vi "Statemachine example.vi"() -> ()   [LabVIEW 2026]
uses:
  statemachine control_1.ctl
panel:
  out "motor on time[ms]":u32
  out "millisecond timer value":u32
  out "motor on":bool
  in  "MOTOR TIMER [ms]":i32
  in  "user button":bool
  in  "index pulse":bool
  out "State":T1
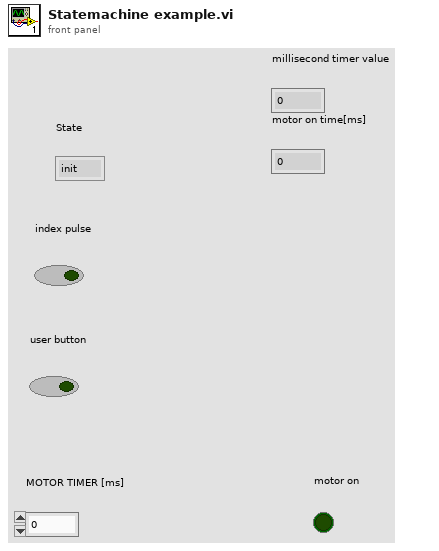
[diagram p1: front panel]
types:
  T1 = typedef "statemachine control_1.ctl" = enum16{"init", "waiting for pulse", "waiting for button", " running motor", "shut down"}
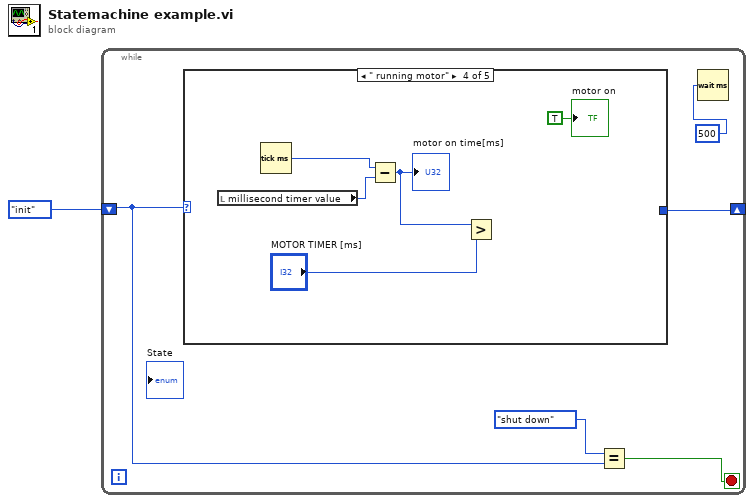
[diagram p0: block diagram]
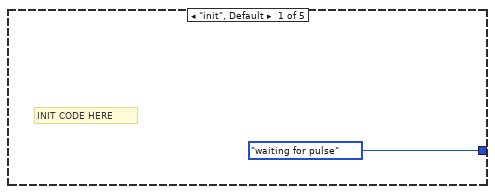
[diagram p2: hidden frame]
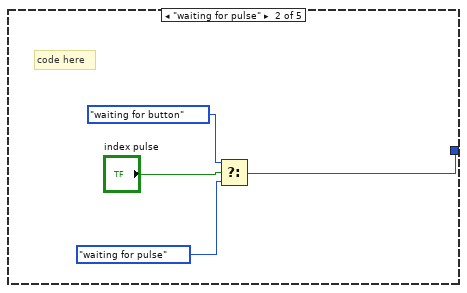
[diagram p3: hidden frame]
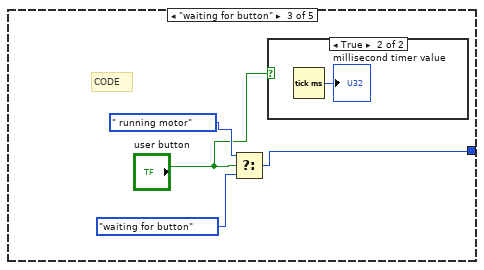
[diagram p4: hidden frame]
diagram:
  n1 = while {
    shift-right: [w6] -> _
    shift-left: statemachine_control_1."init" ("State") -> [w2]
    stop <- w5 stop-if-true
    n2 = case shown="\" running motor\"" w2 {
      tunnel: [statemachine_control_1."waiting for pulse" ("State") w10 w13 _ _] -> w6
      frame "init", Default {
        # "INIT CODE HERE"
      }
      frame "waiting for pulse" {
        # "code here"
        n3 = Select(t=statemachine_control_1."waiting for button" ("State"), s="index pulse", f=statemachine_control_1."waiting for pulse" ("State")) -> (s? t:f=w10:T1)
      }
      frame "waiting for button" {
        # "CODE"
        n4 = Select(t=statemachine_control_1." running motor" ("State"), s="user button", f=statemachine_control_1."waiting for button" ("State")) -> (s? t:f=w13:T1)
        n5 = case shown="True" "user button" {
          frame False {
          }
          frame True {
            n6 = Tick Count (ms)() -> (millisecond timer value=→"millisecond timer value":u32)
          }
        }
      }
      frame " running motor" {
        n7 = local read "millisecond timer value"() -> (w20:u32)
        n8 = Tick Count (ms)() -> (millisecond timer value=w21:u32)
        n9 = Subtract(x=w21, y=w20) -> (x-y=w17:u32)
        "motor on time[ms]" <- w17
        n10 = Greater?(x=w17, y="MOTOR TIMER [ms]") -> ()  [unwired: 1 out]
        "motor on" <- TRUE ("motor on")
      }
      frame "shut down" {
      }
    }
    n11 = Equal?(x=statemachine_control_1."shut down", y=w2) -> (x = y?=w5:bool)
    n12 = Wait (ms)(milliseconds to wait=u32 500) -> ()  [unwired: 1 out]
  }
